vi "Set Sequence Line.vi"(8 "error in (no error)":errorcluster, 10 "Sequence Line":bool[](array[boolean]), 11 "VISA resource name":refnum<visa-resource-name>) -> (0 "error out":errorcluster, 3 "VISA resource name out":refnum<visa-resource-name>)   [LabVIEW 2020, in "QuPMXdriver.lvlib"]
doc: "Enable/disable multiple channels based on a 1D array of booleans (one line of a Sequence). The array address channels in following matter: slave 1 channel 1; slave 1 channel 2; slave 2 channel 1, slave 2 channel 2, slave 3 channel 1 ..."
uses:
  QuPMXdriver.lvlib
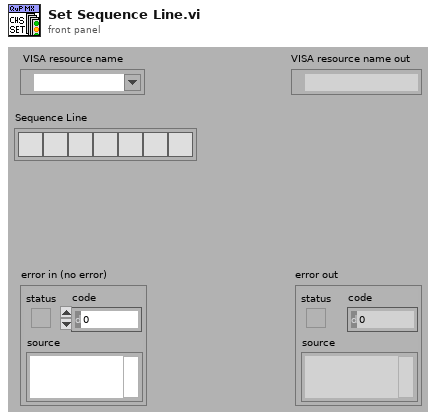
[diagram p1: front panel]
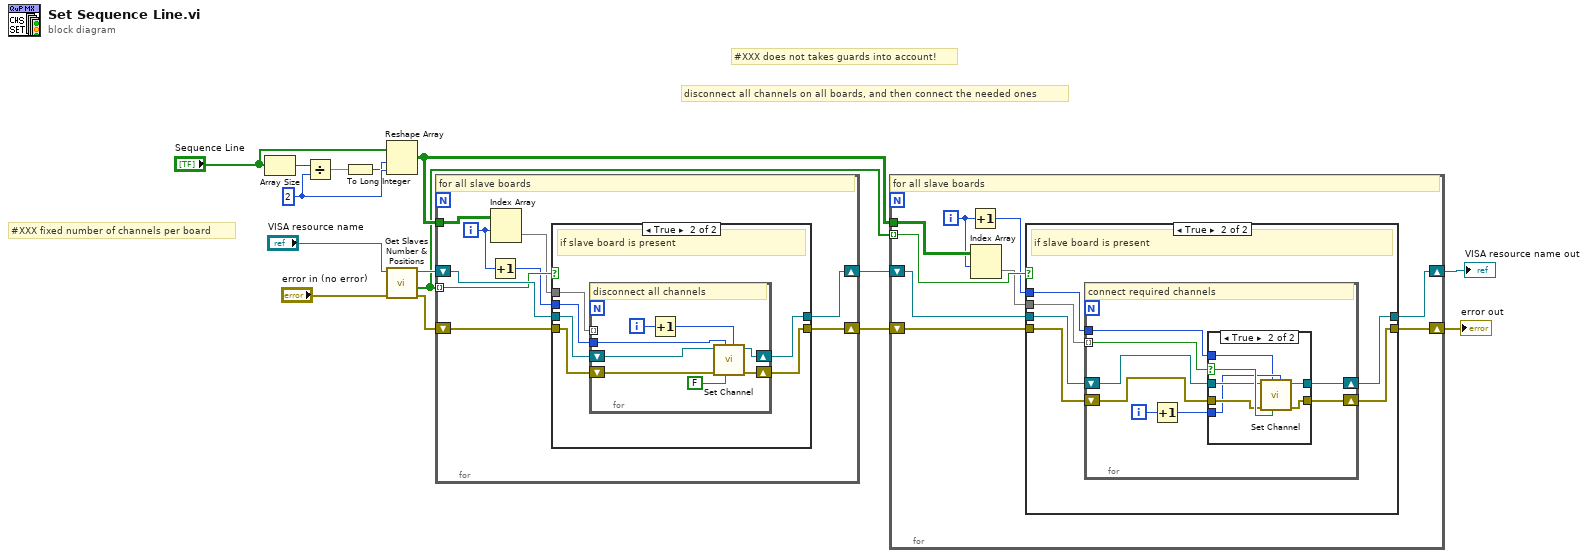
[diagram p0: block diagram]
diagram:
  w12 = 2 ("y")
  # "#XXX does not takes guards into account!"
  # "disconnect all channels on all boards, and then connect the needed ones"
  # "#XXX fixed number of channels per board"
  n1 = Array Size(array="Sequence Line") -> (size(s)=w13:i32)
  n2 = Divide(x=w13, y=w12) -> (x/y=w2:dbl)
  n3 = To Long Integer(number=w2) -> (32bit integer=w1:i32)
  n4 = Reshape Array("Sequence Line", w1, w12) -> (w4:bool[][])
  n5 = call "Get Slaves Number & Positions.vi"("error in (no error)"="error in (no error)", "VISA resource name"="VISA resource name") -> ("error out"=w11:errorcluster, "Connected Slaves"=w3:bool[], "VISA resource name out"=w10:refnum<visa-resource-name>)  [unwired: 6 in, 1 out]
  n6 = for {
    tunnel: w4 -> [w19]
    shift-right: [w24] -> w8
    shift-left: w10 -> [w22]
    shift-right: [w21] -> w7
    shift-left: w11 -> [w23]
    tunnel: w3 -> [w20] mode=indexing
    i -> [w18]
    # "for all slave boards"
    n7 = Increment(x=w18) -> (x+1=w17:i32)
    n8 = Index Array(array=w19, index (row)=w18) -> (element=w16:bool[])  [unwired: 1 in]
    n9 = case shown="True" w20 {
      tunnel: w16 -> [_ w29]
      tunnel: [w25 w28] -> w24
      tunnel: w23 -> [w26 w32]
      tunnel: w22 -> [w25 w31]
      tunnel: [w26 w27] -> w21
      tunnel: w17 -> [_ w30]
      frame False {
      }
      frame True {
        # "if slave board is present"
        n10 = for {
          shift-right: [w39] -> w27
          shift-left: w32 -> [w40]
          shift-right: [w37] -> w28
          shift-left: w31 -> [w38]
          tunnel: w30 -> [w33]
          tunnel: w29 -> [_] mode=indexing
          i -> [w35]
          # "disconnect all channels"
          n11 = Increment(x=w35) -> (x+1=w34:i32)
          n12 = call "Set Channel.vi"("Channel"=w34, "Channel Status"=FALSE, "Slave"=w33, "error in (no error)"=w40, "VISA resource name"=w38) -> ("error out"=w39:errorcluster, "VISA resource name out"=w37:refnum<visa-resource-name>)  [unwired: 5 in]
        }
      }
    }
  }
  n13 = for {
    tunnel: w4 -> [w44]
    shift-right: [w49] -> w6
    shift-left: w8 -> [w47]
    shift-right: [w46] -> w5
    shift-left: w7 -> [w48]
    tunnel: w3 -> [w45] mode=indexing
    i -> [w43]
    # "for all slave boards"
    n14 = Increment(x=w43) -> (x+1=w42:i32)
    n15 = Index Array(array=w44, index (row)=w43) -> (element=w41:bool[])  [unwired: 1 in]
    n16 = case shown="True" w45 {
      tunnel: w41 -> [_ w54]
      tunnel: [w50 w57] -> w49
      tunnel: w48 -> [w51 w52]
      tunnel: w47 -> [w50 w53]
      tunnel: [w51 w56] -> w46
      tunnel: w42 -> [_ w55]
      frame False {
      }
      frame True {
        # "if slave board is present"
        n17 = for {
          tunnel: w54 -> [w65] mode=indexing
          shift-right: [w63] -> w56
          shift-left: w52 -> [w64]
          shift-right: [w62] -> w57
          shift-left: w53 -> [w61]
          tunnel: w55 -> [w58]
          i -> [w60]
          # "connect required channels"
          n18 = Increment(x=w60) -> (x+1=w59:i32)
          n19 = case shown="True" w65 {
            selector: w65 -> [_ w74]
            tunnel: w61 -> [w66 w73]
            tunnel: w64 -> [w67 w72]
            tunnel: [w67 w71] -> w63
            tunnel: [w66 w70] -> w62
            tunnel: w59 -> [_ w69]
            tunnel: w58 -> [_ w68]
            frame False {
            }
            frame True {
              n20 = call "Set Channel.vi"("Channel"=w69, "Channel Status"=w74, "Slave"=w68, "error in (no error)"=w72, "VISA resource name"=w73) -> ("error out"=w71:errorcluster, "VISA resource name out"=w70:refnum<visa-resource-name>)  [unwired: 5 in]
            }
          }
        }
      }
    }
  }
  "error out" <- w5
  "VISA resource name out" <- w6
